vi "LWXPS_PositionerCompensationPostExcitationFrequencyNotchFilterSet.vi"(0 "Positioner Name":string, 1 "XPS Reference IN":refnum<k24>, 5 "Notch Frequency Number":i32, 7 "Notch Frequency":dbl, 9 "Notch Bandwidth":dbl, 11 "Notch Gain":dbl, 12 "LabVIEW error IN":errorcluster) -> (4 "XPS Reference OUT":refnum<k24>, 6 "Returned error code":i32, 8 "XPS Error String":string, 15 "LabVIEW error OUT":errorcluster)   [LabVIEW 2014]
uses:
  D:/XPSQ8_LabView_Library/Development/Source/Dll/Newport.XPS.CommandInterface.dll
  Dll/Newport.XPS.CommandInterface.dll
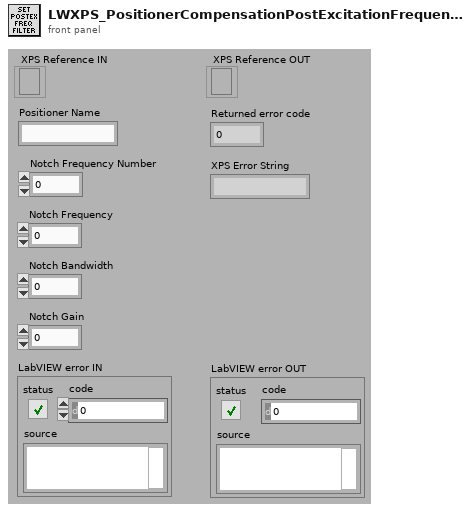
[diagram p1: front panel]
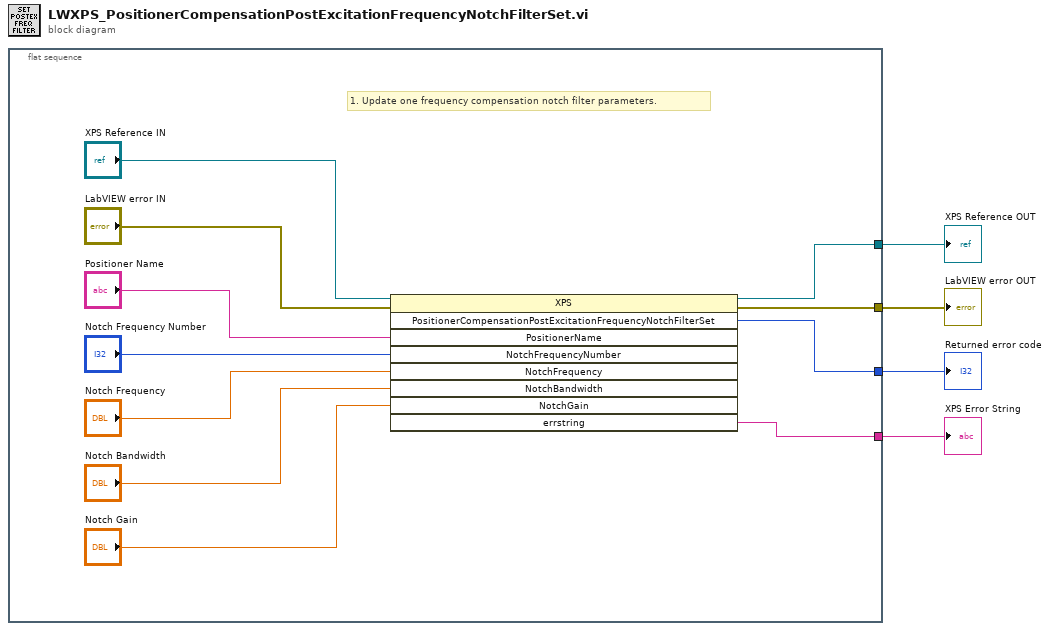
[diagram p0: block diagram]
diagram:
  n1 = flat-sequence {
    tunnel: [w11] -> w4
    tunnel: [w10] -> w3
    tunnel: [w12] -> w2
    tunnel: [w8] -> w1
    frame #0 {
      # "1. Update one frequency compensation notch filter parameters."
      n2 = invoke class="XPS" method="PositionerCompensationPostExcitationFrequencyNotchFilterSet"(reference="XPS Reference IN", error in="LabVIEW error IN", "PositionerName"="Positioner Name", "NotchFrequencyNumber"="Notch Frequency Number", "NotchFrequency"="Notch Frequency", "NotchBandwidth"="Notch Bandwidth", "NotchGain"="Notch Gain") -> (reference out=w11:refnum<k24>, error out=w10:errorcluster, "PositionerCompensationPostExcitationFrequencyNotchFilterSet"=w12:i32, "errstring"=w8:string)  [unwired: 2 in, 5 out]
    }
  }
  "XPS Error String" <- w1
  "XPS Reference OUT" <- w4
  "LabVIEW error OUT" <- w3
  "Returned error code" <- w2
